vi "Global - Configuration Options.vi"() -> ()   [LabVIEW 2013]
panel:
  in  "Error Log Duplicate Interval (ms)":u32=5000
  in  "Network Stream Polling Timeout (ms)":i32=500
  in  "Debugging":bool=TRUE
  in  "Error Log Max Size (bytes)":i64=100000
  in  "RT Error Log":path=path "c:/logs/log.txt"
  in  "Control Period (ticks)":u32=40000
  in  "Timeout Period (ticks)":u64=40000000
  in  "RT Stream Name":string="Command Stream from RT"
  in  "Monitoring Loop Rate (ms)":u32=200
  in  "Watchdog Pet Rate (ms)":u32=100
  in  "UI Stream Name":string="Command Stream from UI"
  in  "Network Stream Connect Timeout (ms)":i32=5000
  # "If you change any of these default configuration options, you must select Edit > Make Current Values Default before saving this VI."
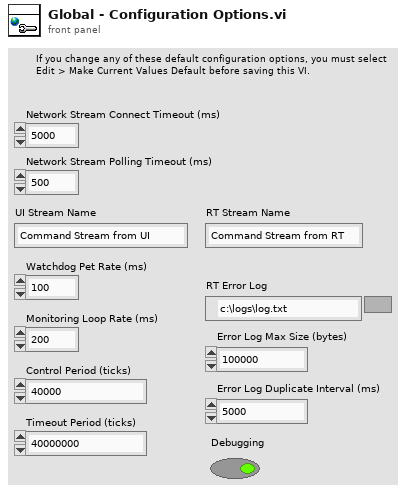
[diagram p1: front panel]
diagram:
